vi "Copy Images to Outut Dir.vi"(8 "error in (no error)":errorcluster, 11 "Parse Presentation in":refnum<class "Parse Presentation.lvclass">) -> (0 "error out":errorcluster, 3 "Parse Presentation out":refnum<class "Parse Presentation.lvclass">)   [LabVIEW 2015, in "Parse Presentation.lvclass"]
uses:
  Parse Presentation.lvclass
  Parse Presentation.lvclass/Parse Presentation.ctl
  <vilib>/regexp/Match Regular Expression.xnode
  <vilib>/zip/NI_Unzip.lvlib
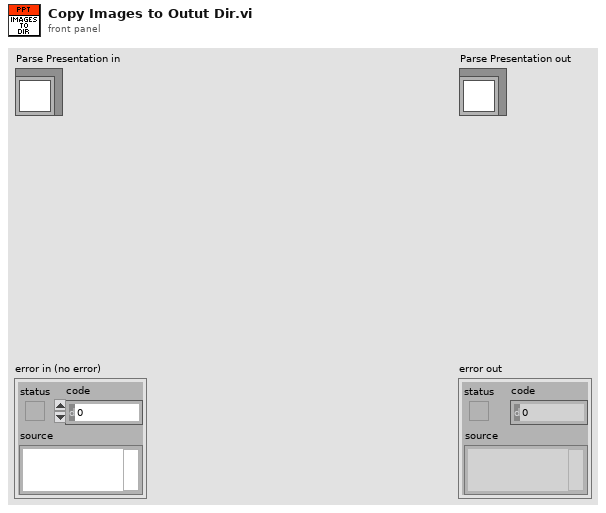
[diagram p1: front panel]
types:
  T1 = typedef "Parse Presentation.lvclass/Slide Info..cluster.ctl" = cluster{"Slide":i32, "Text":string, "Images":string}
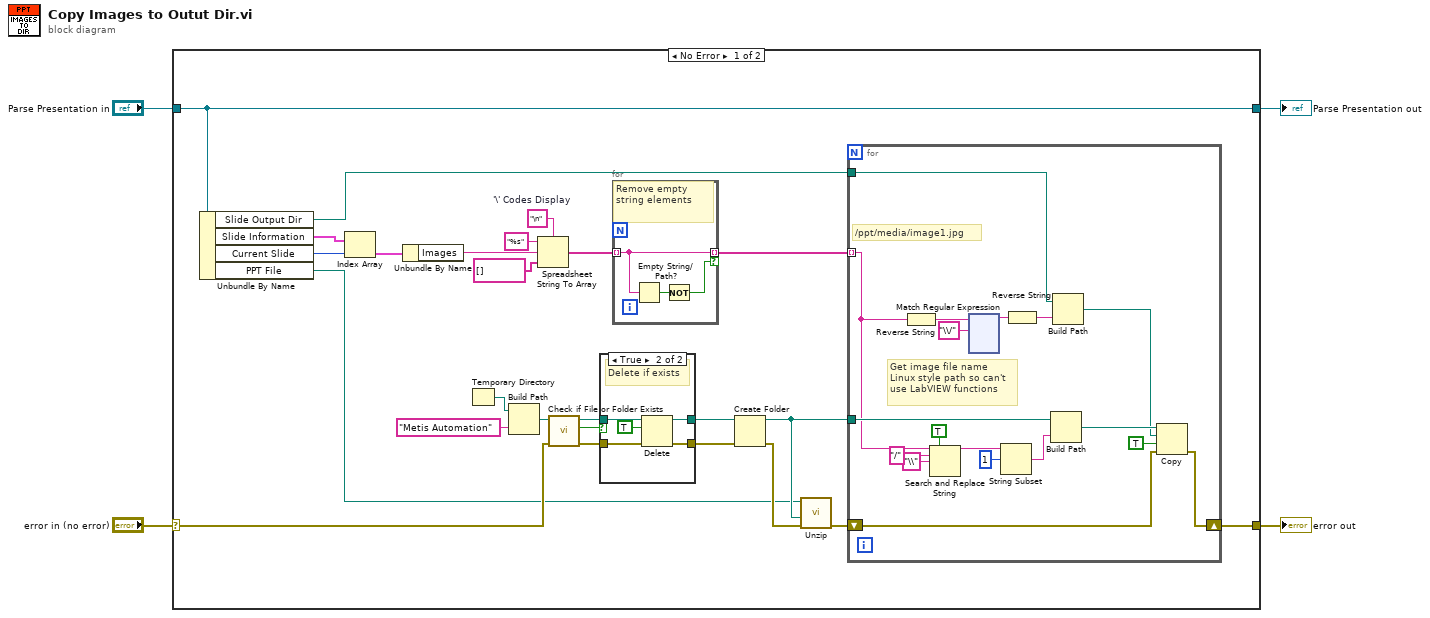
[diagram p0: block diagram]
diagram:
  n1 = case shown="No Error" "error in (no error)" {
    selector: "error in (no error)" -> [w11 w173]
    tunnel: [w12 w173] -> w3
    tunnel: [w10 w172] -> w1
    tunnel: "Parse Presentation in" -> [w10 w172]
    frame No Error {
      w15 = "\n"  # '\' Codes Display
      n2 = Unbundle By Name(w10) -> ("Slide Output Dir"=w6:path, "Slide Information"=w9:T1[], "Current Slide"=w8:i32, "PPT File"=w5:path)
      n3 = Index Array(array=w9, index=w8) -> (element=w7:T1)
      n4 = Unbundle By Name(w7) -> ("Images"=w13:string)
      n5 = Temporary Directory() -> (w26:path)
      n6 = Build Path(base path=w26, name or relative path="Metis Automation") -> (appended path=w24:path)
      n7 = Spreadsheet String To Array(delimiter (Tab)=w15, format string="%s", spreadsheet string=w13, array type (2D Dbl)=string[] []) -> (array=w17:string[])
      n8 = call <vilib>:"Check if File or Folder Exists.vi"("error in (no error)"=w11, "path"=w24) -> ("error out"=w21:errorcluster, "file or folder exists?"=w22:bool, "dup path"=w23:path)  [unwired: 7 in]
      n9 = case shown="True" w22 {
        tunnel: w23 -> [w162 w168]
        tunnel: w21 -> [w163 w167]
        tunnel: [w163 w166] -> w19
        tunnel: [w162 w165] -> w20
        frame False {
        }
        frame True {
          # "Delete if exists"
          n10 = Delete(path (use dialog)=w168, entire hierarchy (F)=TRUE, error in=w167) -> (deleted path=w165:path, error out=w166:errorcluster)  [unwired: 2 in, 1 out]
        }
      }
      n11 = for {
        tunnel: w17 -> [w170] mode=indexing
        tunnel: [w170] -> w27 mode=indexing if=w169
        # "Remove empty string elements"
        n12 = Empty String/Path?(string/path=w170) -> (empty?=w171:bool)
        n13 = Not(x=w171) -> (.not. x?=w169:bool)
      }
      n14 = Create Folder(path (use dialog)=w20, error in=w19) -> (created path=w28:path, error out=w18:errorcluster)  [unwired: 1 in, 1 out]
      n15 = call <vilib>:"Unzip.vi"("error in (no error)"=w18, "Target directory (same as Zip file if empty)"=w28, "Zip file"=w5) -> ("error out"=w29:errorcluster)  [unwired: 6 in, 2 out]
      n16 = for {
        tunnel: w27 -> [w41] mode=indexing
        tunnel: w28 -> [w47]
        tunnel: w6 -> [w46]
        shift-right: [w30] -> w12
        shift-left: w29 -> [w31]
        # "Get image file name\nLinux style path so can't\nuse LabVIEW functions"
        # "/ppt/media/image1.jpg"
        n17 = Reverse String(1:w41) -> (0:w45:string)
        n18 = Search and Replace String(replace all?=TRUE ("replace all? (F)"), input string=w41, search string="/", replace string="\\" ("replace string (\"\")")) -> (result string=w36:string)  [unwired: 4 in, 3 out]
        n19 = xnode "Match Regular Expression"("input string"=w45, "regular expression"="\\/") -> ("before match"=w43:string)  [unwired: 4 in, 4 out]
        n20 = String Subset(string=w36, offset (0)=1) -> (substring=w35:string)  [unwired: 1 in]
        n21 = Reverse String(1:w43) -> (0:w42:string)
        n22 = Build Path(base path=w47, name or relative path=w35) -> (appended path=w34:path)
        n23 = Build Path(base path=w46, name or relative path=w42) -> (appended path=w33:path)
        n24 = Copy(8:w31, 9:TRUE ("overwrite (F)"), 10:w33, 11:w34) -> (0:w30:errorcluster)  [unwired: 1 in, 2 out]
      }
    }
    frame Error {
    }
  }
  "error out" <- w3
  "Parse Presentation out" <- w1
